vi "TDC_init.vi"(8 "Error In":errorcluster, 11 "Device ID":i32) -> (0 "Error Out":errorcluster)   [LabVIEW 2013]
uses:
  lib/tdcbase.dll
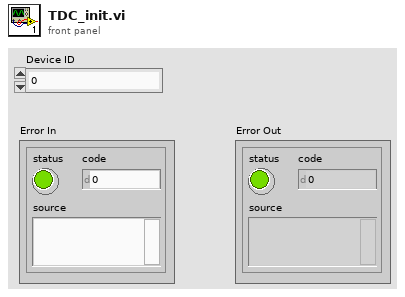
[diagram p1: front panel]
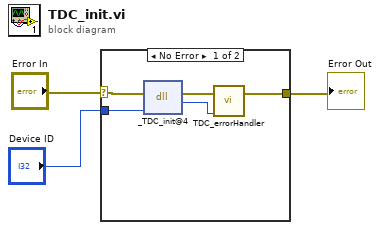
[diagram p0: block diagram]
diagram:
  n1 = case shown="No Error" "Error In" {
    selector: "Error In" -> [w8 w9]
    tunnel: [w6 w9] -> w2
    tunnel: "Device ID" -> [w4 _]
    frame No Error {
      n2 = dll-call lib="C:/Users/science/Desktop/NVExperimeent/Labview/QUTAU-15_06_25/userlib/lib/tdcbase.dll" fn="_TDC_init@4"(error in=w8, "deviceId"=w4) -> (error out=w7:errorcluster, "return type"=w5:i32)  [unwired: 3 in, 1 out]
      n3 = call "TDC_errorHandler.vi"("quTAU Return Code"=w5, "Error In"=w7) -> ("Error Out"=w6:errorcluster)  [unwired: 9 in]
    }
    frame Error {
    }
  }
  "Error Out" <- w2
